vi "pressure calibration.vi"(11 "input variable":dbl) -> (3 "output variable":dbl)   [LabVIEW 2020]
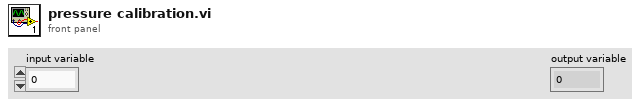
[diagram p1: front panel]
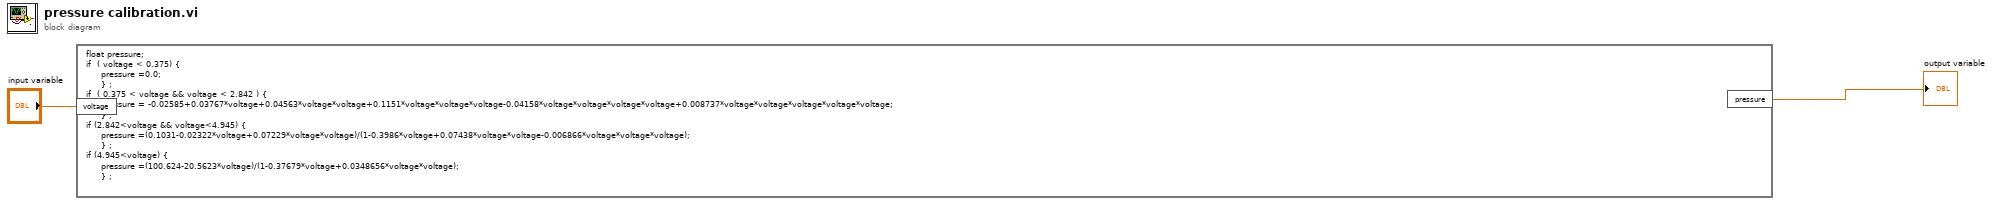
[diagram p0: block diagram]
diagram:
  n1 = formula code="float pressure;\nif  ( voltage < 0.375) {\n     pressure =0.0;\n     } ;\nif  ( 0.375 < voltage && voltage < 2.842 ) {\n     pressure = -0.02585+0.03767*voltage+0.04563*voltage*voltage+0.1151*voltage*voltage*voltage-0.04158*voltage*voltage*voltage*voltage+0.008737*voltage*voltage*voltage*voltage*voltage;\n     } ;\nif (2.842<voltage && voltage<4.945) {\n     pressure =(0.1031-0.02322*voltage+0.07229*voltage*voltage)/(1-0.3986*voltage+0.07438*voltage*voltage-0.006866*voltage*voltage*voltage);\n     } ;\nif (4.945<voltage) {\n     pressure =(100.624-20.5623*voltage)/(1-0.37679*voltage+0.0348656*voltage*voltage);\n     } ;"("voltage"="input variable") -> ("pressure"=→"output variable":dbl)
